vi "RelativeMove.vi"(0 "CmdLib In":refnum<k24>, 1 "DeviceKey In":string, 2 "Device Address In":i32, 3 "Motor":i32, 4 "Relative Steps":i32, 5 "error in (no error)":errorcluster) -> (14 "CmdLib Out":refnum<k24>, 16 "DeviceKey Out":string, 17 "Device Address Out":i32, 19 "error out":errorcluster)   [LabVIEW 2013]
uses:
  C:/GEECS/Developers Version/source/Device Driver/Picomotor8742dotNet/NewFocus/CmdLib.dll
  CmdLib.dll
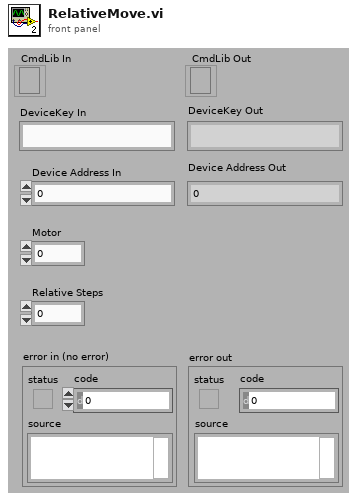
[diagram p1: front panel]
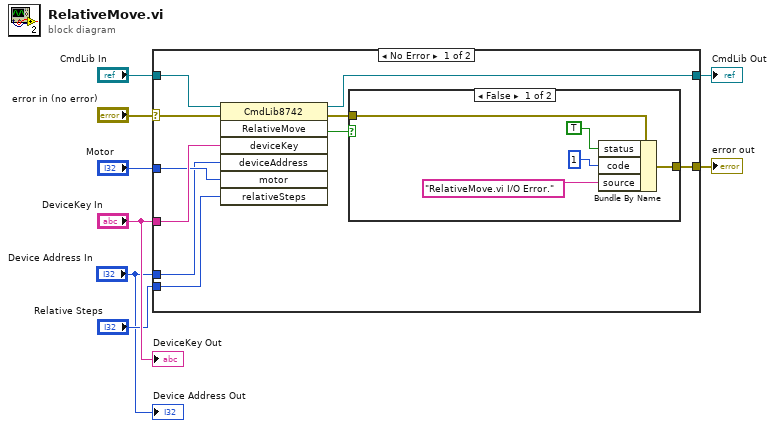
[diagram p0: block diagram]
diagram:
  n1 = case shown="No Error" "error in (no error)" {
    selector: "error in (no error)" -> [w15 w25]
    tunnel: "CmdLib In" -> [w18 w26]
    tunnel: [w17 w26] -> w7
    tunnel: "Motor" -> [w10 _]
    tunnel: "DeviceKey In" -> [w16 _]
    tunnel: [w12 w25] -> w4
    tunnel: "Relative Steps" -> [w11 _]
    tunnel: "Device Address In" -> [w9 _]
    frame No Error {
      n2 = invoke class="CmdLib8742" method="RelativeMove"(reference=w18, error in=w15, "deviceKey"=w16, "deviceAddress"=w9, "motor"=w10, "relativeSteps"=w11) -> (reference out=w17:refnum<k24>, error out=w13:errorcluster, "RelativeMove"=w14:bool)  [unwired: 1 in, 4 out]
      n3 = case shown="False" w14 {
        tunnel: w13 -> [w23 w24]
        tunnel: [w22 w24] -> w12
        frame False {
          n4 = Bundle By Name(cluster=w23, "status"=TRUE, "code"=1, "source"="RelativeMove.vi I/O Error.") -> (w22:errorcluster)
        }
        frame True {
        }
      }
    }
    frame Error {
    }
  }
  "error out" <- w4
  "CmdLib Out" <- w7
  "DeviceKey Out" <- "DeviceKey In"
  "Device Address Out" <- "Device Address In"
